vi "Send Time Stamp.vi"(10 "Time session in":refnum<k21>, 11 "Refnum in":refnum<k21>) -> (0 "error out":errorcluster)   [LabVIEW 2014]
uses:
  <vilib>/xnet/xnet.llb/XNET Frame CAN.ctl
  <vilib>/xnet/xnet.llb/XNET Frame Type CAN.ctl
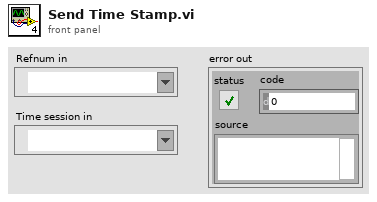
[diagram p1: front panel]
types:
  T1 = typedef "XNET Frame Type CAN.ctl" = u8
  T2 = typedef "XNET Frame CAN.ctl" = cluster{"timestamp":timestamp, "payload":u8[], "identifier":u32, "type":T1, "extended?":bool, "echo?":bool}
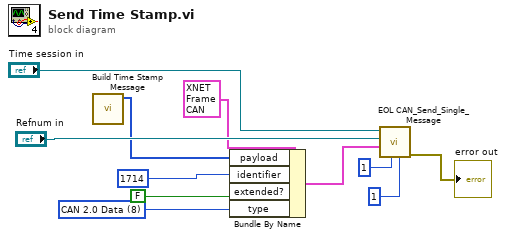
[diagram p0: block diagram]
diagram:
  w5 = T1 8 items=["CAN Data"=0, "CAN Remote"=1, "CAN Bus Error"=2, "CAN 2.0 Data"=8, "CAN FD Data"=16, "CAN FD+BRS Data"=24, "J1939 Data"=192, "Delay"=224, "Log Trigger"=225, "Start Trigger"=226] ("type")
  n1 = call "Build Time Stamp Message.vi"() -> ("Array"=w2:u32[])  [unwired: 11 in]
  n2 = Bundle By Name(cluster=T2 {"timestamp"=timestamp(0 s since 1904-01-01), "payload"=[2, 39, 3, 85, 85, 85, 85, 85], "identifier"=402391172, "type"=0, "extended?"=TRUE, "echo?"=FALSE} ("Tx CAN frame"), "payload"=w2, "identifier"=u32 1714, "extended?"=FALSE, "type"=w5) -> (w11:T2)
  n3 = call "EOL CAN_Send_Single_Message.vi"("Retries"=1, "Msg Wait Time"=u32 1, "Tx CAN frame"=w11, "Read Session in"="Refnum in", "Write Session in"="Time session in") -> ("Error out"=→"error out":errorcluster)  [unwired: 2 in, 4 out]
